vi "VICI Reserve Pump.vi"(8 "error in (no error)":errorcluster, 10 "Pump ID":string, 11 "VISA # in":string) -> (0 "error out":errorcluster, 2 "Loop Completed":bool, 3 "VISA # out":string)   [LabVIEW 2018, in "VICI M6 M50 Party Mode.lvlib" / "VICI Global Library.lvlib"]
uses:
  VICI Global Library.lvlib
  VICI Global Array.ctl
  VICI Global.ctl
panel:
  out "Boolean":bool
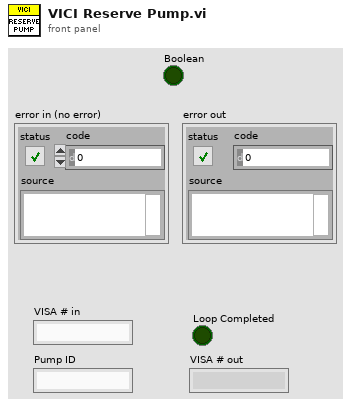
[diagram p1: front panel]
types:
  T1 = typedef "VICI M6 M50 Party Mode.lvlib/VICI Global Library.lvlib/VICI Global.ctl" = cluster{"Busy":bool, "VISA #":string, "Current Pump":string, "Pump Array":string[], "Last Success":timestamp, "ID Queue":string[]}
  T2 = typedef "VICI M6 M50 Party Mode.lvlib/VICI Global Library.lvlib/VICI Global Array.ctl" = T1[]
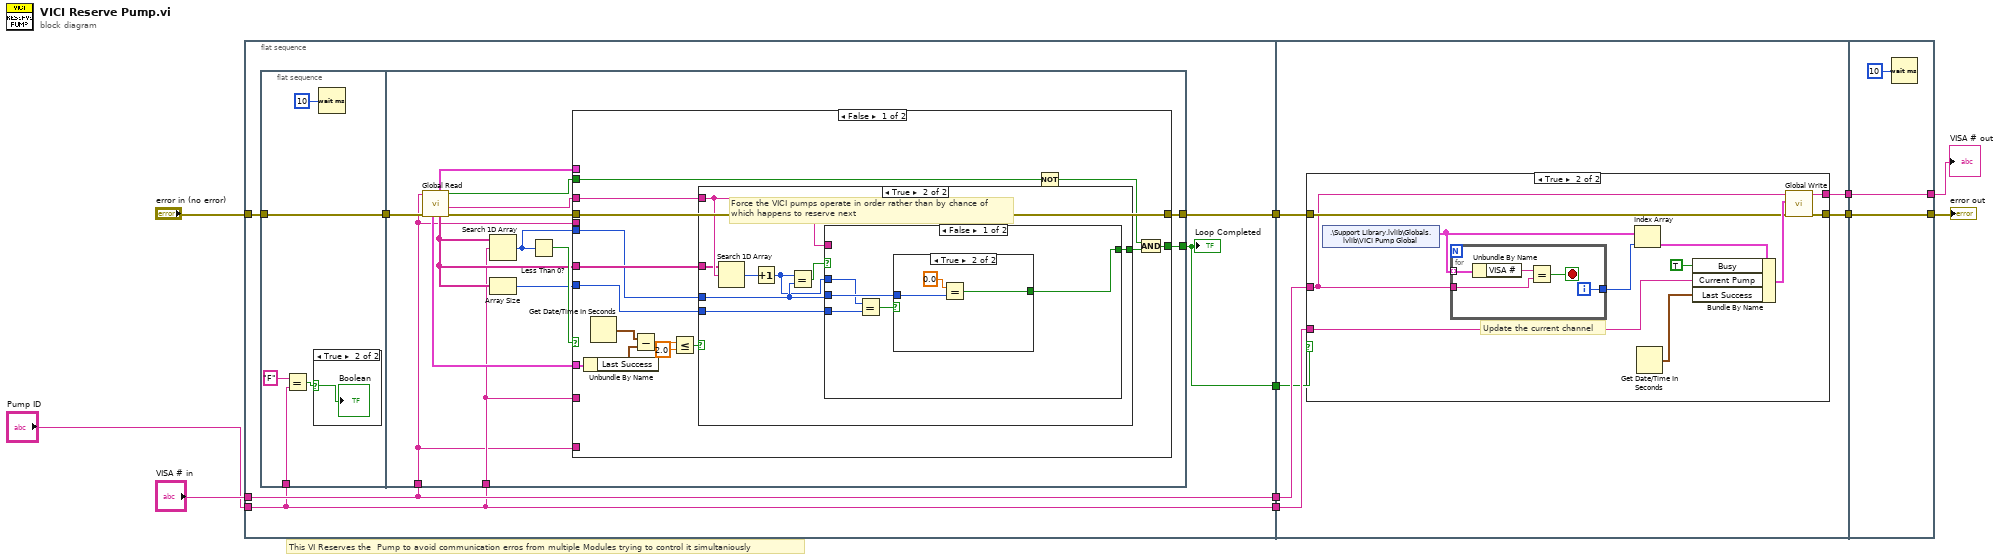
[diagram p0: block diagram]
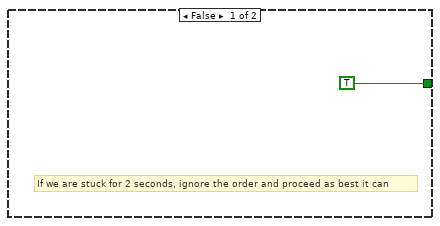
[diagram p3: hidden frame]
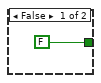
[diagram p4: hidden frame]
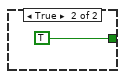
[diagram p5: hidden frame]
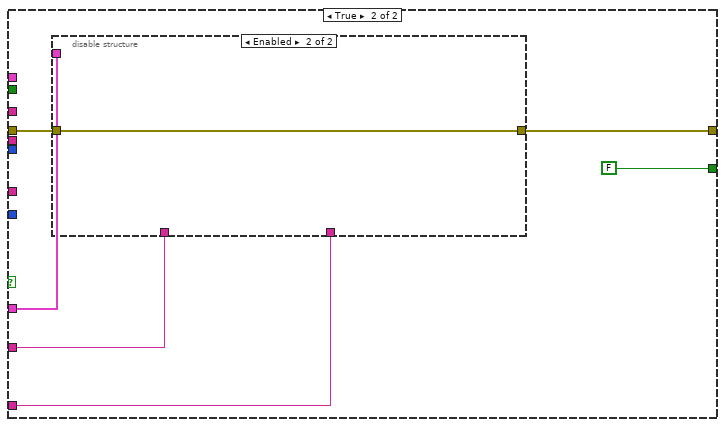
[diagram p6: hidden frame]
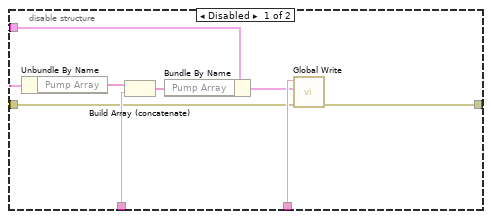
[diagram p7: hidden frame]
diagram:
  # "This VI Reserves the  Pump to avoid communication erros from multiple Modules trying to control it simultaniously"
  n1 = flat-sequence {
    tunnel: [w16] -> w11
    tunnel: [w13] -> w10
    tunnel: "error in (no error)" -> [w17]
    tunnel: [w12] -> w9
    tunnel: "Pump ID" -> [w12]
    tunnel: [w14] -> w8
    tunnel: "VISA # in" -> [w13]
    tunnel: [w91] -> w7
    tunnel: w11 -> [w92]
    tunnel: w10 -> [w90]
    tunnel: w9 -> [w89]
    tunnel: [w88] -> w6
    tunnel: w8 -> [w87]
    tunnel: [w113] -> w5
    tunnel: w7 -> [w113]
    tunnel: [w111] -> w2
    tunnel: w6 -> [w111]
    frame #0 {
      n2 = flat-sequence {
        tunnel: [w22] -> w15
        tunnel: w17 -> [w22]
        tunnel: w12 -> [w19]
        tunnel: [w36] -> w16
        tunnel: [w37] -> w14
        tunnel: w15 -> [w33]
        tunnel: w12 -> [w25]
        tunnel: w13 -> [w24]
        frame #0 {
          n3 = Equal?(x="F", y=w19) -> (x = y?=w20:bool)
          n4 = case shown="True" w20 {
            selector: w20 -> [_ w23]
            frame False {
            }
            frame True {
              "Boolean" <- w23
            }
          }
          n5 = Wait (ms)(milliseconds to wait=u32 10) -> ()  [unwired: 1 out]
        }
        frame #1 {
          n6 = call "Global Read.vi"("VISA #"=w24, "error in (no error)"=w33) -> ("Global for this VISA"=w26:T1, "VICI Global Array Out"=w27:T2, "Pump Array"=w30:string[], "Busy"=w32:bool, "Current Pump"=w31:string, "error out"=w28:errorcluster)  [unwired: 2 in, 1 out]
          n7 = Search 1D Array(1D array=w30, element=w25) -> (index of element=w35:i32)  [unwired: 1 in]
          n8 = Array Size(array=w30) -> (size(s)=w29:i32)
          n9 = Less Than 0?(x=w35) -> (x < 0?=w34:bool)
          n10 = case shown="False" w34 {
            tunnel: w32 -> [w52 _]
            tunnel: [w51 FALSE] -> w37
            tunnel: w28 -> [w50 w74]
            tunnel: [w50 w73] -> w36
            tunnel: w31 -> [w49 _]
            tunnel: w30 -> [w48 _]
            tunnel: w29 -> [w47 _]
            tunnel: w35 -> [w46 _]
            tunnel: w24 -> [_ _]
            tunnel: w27 -> [_ _]
            tunnel: w26 -> [w42 w77]
            tunnel: w25 -> [_ w76]
            tunnel: w24 -> [_ w75]
            frame False {
              n11 = Unbundle By Name(w42) -> ("Last Success"=w41:timestamp)
              n12 = Get Date/Time In Seconds() -> (seconds since 1Jan1904=w43:timestamp)
              n13 = Subtract(x=w43, y=w41) -> (x-y=w40:dbl)
              n14 = Less Or Equal?(x=w40, y=2.0) -> (x <= y?=w38:bool)
              n15 = case shown="True" w38 {
                tunnel: w49 -> [_ w61]
                tunnel: w48 -> [_ w60]
                tunnel: w47 -> [_ w59]
                tunnel: w46 -> [_ w58]
                tunnel: [TRUE w56] -> w44
                frame False {
                  # "If we are stuck for 2 seconds, ignore the order and proceed as best it can"
                }
                frame True {
                  # "Force the VICI pumps operate in order rather than by chance of\nwhich happens to reserve next"
                  n16 = Search 1D Array(1D array=w60, element=w61) -> (index of element=w55:i32)  [unwired: 1 in]
                  n17 = Increment(x=w55) -> (x+1=w54:i32)
                  n18 = Equal?(x=w54, y=w58) -> (x = y?=w57:bool)
                  n19 = case shown="False" w57 {
                    tunnel: [w66 TRUE] -> w56
                    tunnel: w59 -> [w65 _]
                    tunnel: w61 -> [_ _]
                    tunnel: w58 -> [w63 _]
                    tunnel: w54 -> [w62 _]
                    frame False {
                      n20 = Equal?(x=w62, y=w65) -> (x = y?=w64:bool)
                      n21 = case shown="True" w64 {
                        tunnel: [FALSE w68] -> w66
                        tunnel: w63 -> [_ w69]
                        frame False {
                        }
                        frame True {
                          n22 = Equal?(x=0.0, y=w69) -> (x = y?=w68:bool)
                        }
                      }
                    }
                    frame True {
                    }
                  }
                }
              }
              n23 = Not(x=w52) -> (.not. x?=w45:bool)
              n24 = And(x=w45, y=w44) -> (x .and. y?=w51:bool)
            }
            frame True {
              n25 = disable-structure shown="Enabled" {
                disable-tunnel: w77 -> [w85 _]
                disable-tunnel: w76 -> [w84 _]
                disable-tunnel: w75 -> [w83 _]
                disable-tunnel: w74 -> [w82 w86]
                disable-tunnel: [w81 w86] -> w73
                frame Disabled {
                  n26 = Unbundle By Name(w85) -> ("Pump Array"=w80:string[])
                  n27 = Build Array (concatenate)(w80, w84) -> (w79:string[])
                  n28 = Bundle By Name(cluster=w85, "Pump Array"=w79) -> (w78:T1)
                  n29 = call "Global Write.vi"("error in (no error)"=w82, "VICI Global"=w78, "VISA # in"=w83) -> ("error out"=w81:errorcluster)  [unwired: 7 in, 1 out]
                }
                frame Enabled {
                }
              }
            }
          }
        }
      }
      "Loop Completed" <- w14
    }
    frame #1 {
      n30 = case shown="True" w87 {
        tunnel: w92 -> [w94 w98]
        tunnel: [w94 w99] -> w91
        tunnel: w90 -> [w93 w96]
        tunnel: w89 -> [_ w102]
        tunnel: [w93 w97] -> w88
        frame False {
        }
        frame True {
          # "Update the current channel"
          n31 = shared-variable ".\\Support Library.lvlib\\Globals.lvlib\\VICI Pump Global"() -> (w103:T2)  [unwired: 1 in, 1 out]
          n32 = for {
            tunnel: w103 -> [w110] mode=indexing
            tunnel: w96 -> [w108]
            tunnel: [w106] -> w101
            i -> [w106]
            stop <- w107 stop-if-true
            n33 = Unbundle By Name(w110) -> ("VISA #"=w109:string)
            n34 = Equal?(x=w109, y=w108) -> (x = y?=w107:bool)
          }
          n35 = Index Array(array=w103, index=w101) -> (element=w104:T1)
          n36 = Get Date/Time In Seconds() -> (seconds since 1Jan1904=w95:timestamp)
          n37 = Bundle By Name(cluster=w104, "Busy"=TRUE, "Current Pump"=w102, "Last Success"=w95) -> (w100:T1)
          n38 = call "Global Write.vi"("error in (no error)"=w98, "VICI Global"=w100, "VISA # in"=w96) -> ("error out"=w99:errorcluster, "VISA # out"=w97:string)  [unwired: 7 in]
        }
      }
    }
    frame #2 {
      n39 = Wait (ms)(milliseconds to wait=u32 10) -> ()  [unwired: 1 out]
    }
  }
  "error out" <- w5
  "VISA # out" <- w2
